vi "ForceAndReadNew.vi"(0 "object in":refnum<class "CoriFlowBFS1Plus.lvclass">, 2 "Buffer Values":bool=TRUE, 5 "error in (no error)":errorcluster) -> (14 "object out":refnum<class "CoriFlowBFS1Plus.lvclass">, 16 "New Data":T1, 19 "error out":errorcluster)   [LabVIEW 2021, in "CoriFlowBFS1Plus.lvclass"]
uses:
  CoriFlowBFS1Plus.lvclass
  CoriFlowBFS1Plus.lvclass/CoriFlowBFS1Plus.ctl
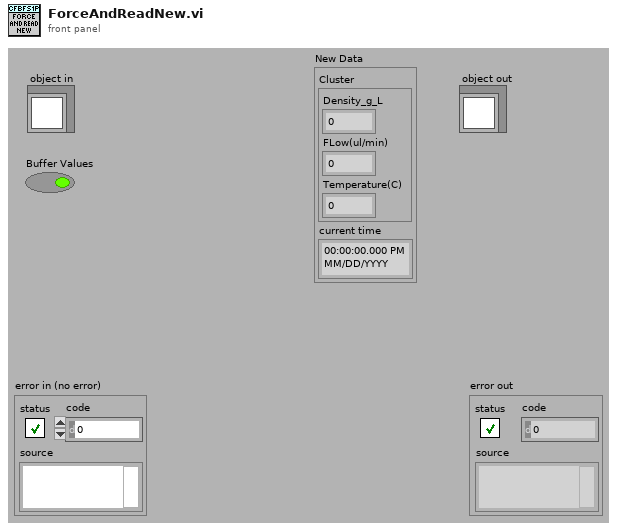
[diagram p1: front panel]
types:
  T1 = cluster{"Cluster":cluster{"Density_g_L":sgl, "FLow(ul/min)":sgl, "Temperature(C)":sgl}, "current time":timestamp}
  T2 = cluster{"Message":string, "Message Data":variant}
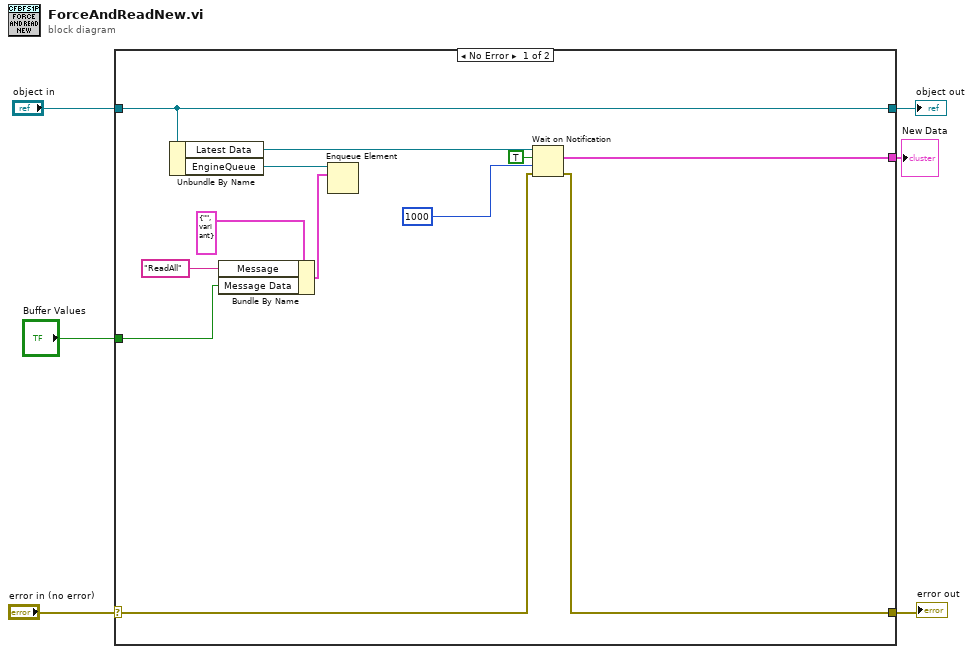
[diagram p0: block diagram]
diagram:
  n1 = case shown="No Error" "error in (no error)" {
    selector: "error in (no error)" -> [w13 w20]
    tunnel: [w12 w20] -> w5
    tunnel: [w18 w19] -> w3
    tunnel: "object in" -> [w18 w19]
    tunnel: [w16 _] -> w2
    tunnel: "Buffer Values" -> [w7 _]
    frame No Error {
      n2 = Unbundle By Name(w18) -> ("Latest Data"=w17:refnum<notifier>, "EngineQueue"=w11:refnum<queue>)
      n3 = Bundle By Name(cluster=T2 {"Message"="", "Message Data"=variant} ("element"), "Message"="ReadAll", "Message Data"=w7) -> (w8:T2)
      n4 = Enqueue Element(queue=w11, element=w8) -> ()  [unwired: 2 in, 3 out]
      n5 = Wait on Notification(notifier=w17, ignore previous (F)=TRUE, timeout in ms (-1)=1000, error in (no error)=w13) -> (notification=w16:T1, error out=w12:errorcluster)  [unwired: 2 out]
    }
    frame Error {
    }
  }
  "error out" <- w5
  "object out" <- w3
  "New Data" <- w2
